vi "Read Trace Data.vi"(5 "Timeout in (0 = OPC timeout)":i32, 7 "Wait for OPC (F)":bool, 8 "error in":errorcluster caption="error in (no error)", 9 "Force ASCII (F)":bool, 10 "Query":string, 11 "VISA session":refnum<visa-resource-name> caption="VISA resource name") -> (0 "error out":errorcluster, 1 "No of Values":i32, 2 "Trace Data":dbl[](array[numeric]) format="%^.3e", 3 "dup VISA session":refnum<visa-resource-name> caption="VISA resource name out")   [LabVIEW 2020, in "Rohde&Schwarz RTx Oscilloscopes.lvlib"]
doc: "This VI reads out trace data from the instrument. It serves as utility VI.\n\nRemote-control command:\nFORMat[:DATA] ASCii | REAL,32"
uses:
  Rohde&Schwarz RTx Oscilloscopes.lvlib
  rsidr_core.lvlib
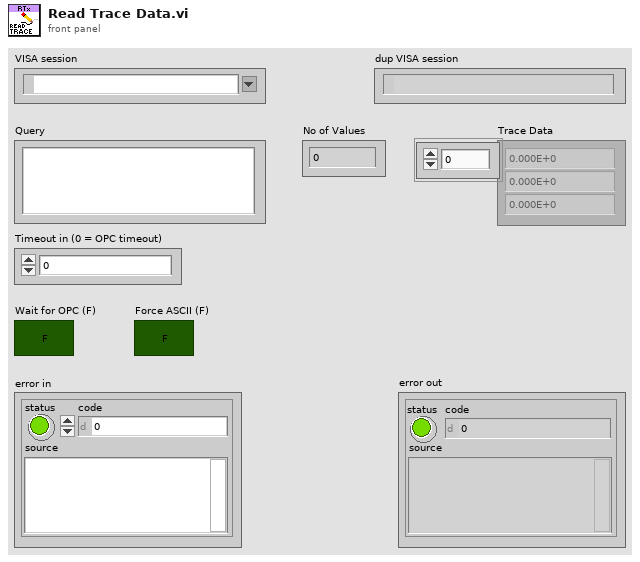
[diagram p1: front panel]
types:
  T1 = typedef "Rohde&Schwarz RTx Oscilloscopes.lvlib/rsidr_core.lvlib/type_Session_Data.ctl" = cluster{"IDN string":string, "Instrument FW":string, "Instr type":string, "Instr type for err. msg.":string, "Installed Options":string[], "Ignore Error Messages":string, "Logging params":variant, "OPC Timeout":i32, "VISA Timeout":i32, "STB Poll VISA Timeout":i32, "Additional Flags":i32, "Wait Before Read":i32, "Wait Before Write":i32, "Option String Flags":i32, "IO Segment Size":i64, "VISA Access Mode":T2, "Interface Type":T3, "OPC Wait Mode":T4, "Bin Float Number  Format":T5, "Bin Integer Number Format":T6, "Simulate":bool, "VXIcapable":bool, "Duplicate Session":bool, "Add LF to Write":bool, "Logging":bool, "Fast Sweep":bool, "Query Instrument Status":bool, "Check Range":bool, "Check Options":bool, "OPC-sync Attr Writes":bool, "OPC-sync Attr Queries":bool}
  T2 = typedef "Rohde&Schwarz RTx Oscilloscopes.lvlib/rsidr_core.lvlib/type_VisaAccessMode.ctl" = u16
  T3 = typedef "Rohde&Schwarz RTx Oscilloscopes.lvlib/rsidr_core.lvlib/type_InterfaceType.ctl" = enum16{"Unknown", "GPIB", "VXI", "GPIB_VXI", "ASRL", "PXI", "TCPIP", "USB", "SOCKET"}
  T4 = typedef "Rohde&Schwarz RTx Oscilloscopes.lvlib/rsidr_core.lvlib/type_OPC_Wait_Mode.ctl" = enum16{"STBpolling", "STBpollingSlow", "STBpollingSuperSlow", "ServiceRequest", "OPCquery"}
  T5 = typedef "Rohde&Schwarz RTx Oscilloscopes.lvlib/rsidr_core.lvlib/type_Binary_Float_Number_Format.ctl" = enum16{"Float_4_Bytes_Swapped", "Float_4_Bytes", "Double_8_Bytes_Swapped", "Double_8_Bytes"}
  T6 = typedef "Rohde&Schwarz RTx Oscilloscopes.lvlib/rsidr_core.lvlib/type_Binary_Integer_Number_Format.ctl" = enum16{"Int32_4_Bytes_Swapped", "Int32_4 Bytes", "Int16_2_Bytes_Swapped", "Int16_2_Bytes"}
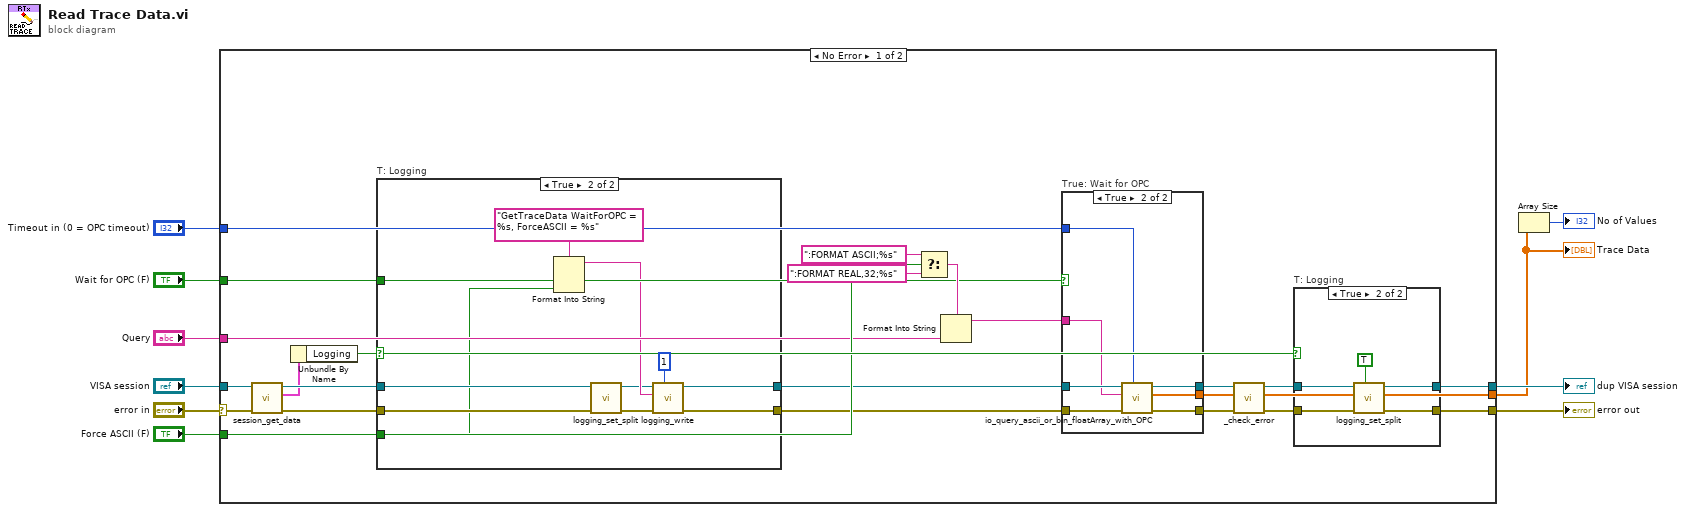
[diagram p0: block diagram]
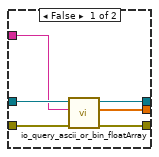
[diagram p2: hidden frame]
diagram:
  n1 = case shown="No Error" "error in" {
    selector: "error in" -> [w33 w68]
    tunnel: [w11 _] -> w3
    tunnel: "Query" -> [w13 _]
    tunnel: "Wait for OPC (F)" -> [w18 _]
    tunnel: "Force ASCII (F)" -> [w20 _]
    tunnel: "VISA session" -> [w32 w67]
    tunnel: [w25 w68] -> w5
    tunnel: [w24 w67] -> w4
    tunnel: "Timeout in (0 = OPC timeout)" -> [w12 _]
    frame No Error {
      n2 = call "session_get_data.vi"("error in"=w33, "VISA resource name"=w32) -> ("error out"=w31:errorcluster, "Session User Data out"=w26:T1, "VISA resource name out"=w30:refnum<visa-resource-name>)  [unwired: 6 in, 1 out]
      n3 = Unbundle By Name(w26) -> ("Logging"=w27:bool)
      n4 = case "T: Logging" shown="True" w27 {
        tunnel: w31 -> [w55 w62]
        tunnel: [w55 w58] -> w16
        tunnel: w30 -> [w54 w61]
        tunnel: [w54 w57] -> w19
        tunnel: w18 -> [_ w63]
        tunnel: w20 -> [_ w56]
        frame False {
        }
        frame True {
          n5 = Format Into String(format string="GetTraceData WaitForOPC = %s, ForceASCII = %s", w63, w56) -> (resulting string=w66:string)  [unwired: 2 in, 1 out]
          n6 = call "logging_set_split.vi"("error in"=w62, "VISA resource name"=w61) -> ("error out"=w60:errorcluster, "VISA resource name out"=w59:refnum<visa-resource-name>)  [unwired: 8 in]
          n7 = call "logging_write.vi"("Add call chain offset\n(No call chain)"=1 ("Add call chain offset\n(No call chain)"), "error in"=w60, "String to write"=w66, "VISA resource name"=w59) -> ("error out"=w58:errorcluster, "VISA resource name out"=w57:refnum<visa-resource-name>)  [unwired: 6 in]
        }
      }
      n8 = Select(t=":FORMAT ASCII;%s", s=w20, f=":FORMAT REAL,32;%s") -> (s? t:f=w21:string)
      n9 = Format Into String(format string=w21, w13) -> (resulting string=w17:string)  [unwired: 2 in, 1 out]
      n10 = case "True: Wait for OPC" shown="True" w18 {
        tunnel: w16 -> [w39 w46]
        tunnel: w19 -> [w38 w45]
        tunnel: [w37 w44] -> w15
        tunnel: [w36 w43] -> w14
        tunnel: w17 -> [w35 w42]
        tunnel: [w34 w41] -> w11
        tunnel: w12 -> [_ w40]
        frame False {
          n11 = call "io_query_ascii_or_bin_floatArray.vi"("error in"=w39, "Query"=w35, "VISA resource name"=w38) -> ("error out"=w37:errorcluster, "Numbers out"=w34:dbl[], "VISA resource name out"=w36:refnum<visa-resource-name>)  [unwired: 5 in, 1 out]
        }
        frame True {
          n12 = call "io_query_ascii_or_bin_floatArray_with_OPC.vi"("Timeout in (0 = OPC timeout)"=w40, "error in"=w46, "Query"=w42, "VISA resource name"=w45) -> ("error out"=w44:errorcluster, "Numbers out"=w41:dbl[], "VISA resource name out"=w43:refnum<visa-resource-name>)  [unwired: 4 in, 1 out]
        }
      }
      n13 = call "_check_error.vi"("error in"=w15, "VISA resource name"=w14) -> ("error out"=w28:errorcluster, "VISA resource name out"=w29:refnum<visa-resource-name>)  [unwired: 8 in]
      n14 = case "T: Logging" shown="True" w27 {
        tunnel: w28 -> [w48 w53]
        tunnel: [w48 w51] -> w25
        tunnel: w29 -> [w47 w52]
        tunnel: [w47 w50] -> w24
        frame False {
        }
        frame True {
          n15 = call "logging_set_split.vi"("Evaluate section error (F)"=TRUE, "error in"=w53, "VISA resource name"=w52) -> ("error out"=w51:errorcluster, "VISA resource name out"=w50:refnum<visa-resource-name>)  [unwired: 7 in]
        }
      }
    }
    frame Error {
    }
  }
  "error out" <- w5
  "dup VISA session" <- w4
  "Trace Data" <- w3
  n16 = Array Size(array=w3) -> (size(s)=→"No of Values":i32)
